vi "LED Shift Step.vi"(10 "LED Interpolate In":T1) -> (0 "Done":bool, 2 "LED Bit Array":u8[](array[numeric]), 3 "LED Interpolate Out":T1)   [LabVIEW 2014]
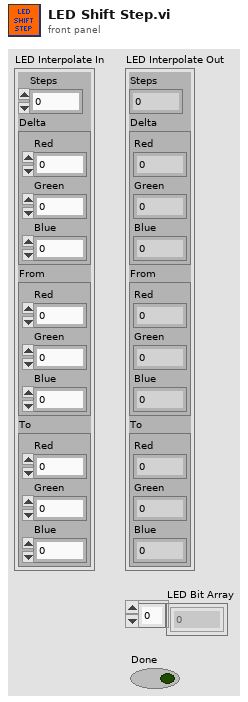
[diagram p1: front panel]
types:
  T1 = cluster{"Steps":i32, "Delta":cluster{"Red":dbl, "Green":dbl, "Blue":dbl}, "From":cluster{"Red":dbl, "Green":dbl, "Blue":dbl}, "To":cluster{"Red":dbl, "Green":dbl, "Blue":dbl}}
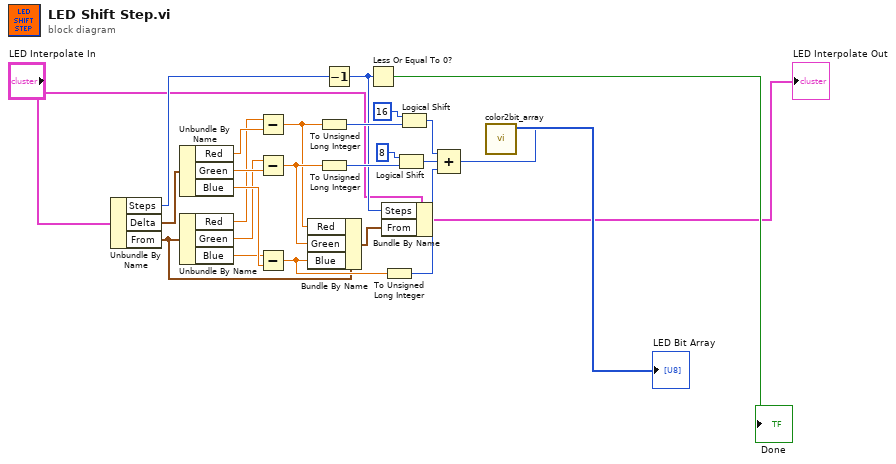
[diagram p0: block diagram]
diagram:
  n1 = Unbundle By Name("LED Interpolate In") -> ("Steps"=w3:i32, "Delta"=w7:cluster{"Red":dbl, "Green":dbl, "Blue":dbl}, "From"=w6:cluster{"Red":dbl, "Green":dbl, "Blue":dbl})
  n2 = Unbundle By Name(w7) -> ("Red"=w9:dbl, "Green"=w11:dbl, "Blue"=w13:dbl)
  n3 = Unbundle By Name(w6) -> ("Red"=w8:dbl, "Green"=w10:dbl, "Blue"=w12:dbl)
  n4 = Subtract(x=w8, y=w9) -> (x-y=w14:dbl)
  n5 = Subtract(x=w10, y=w11) -> (x-y=w20:dbl)
  n6 = Subtract(x=w12, y=w13) -> (x-y=w22:dbl)
  n7 = Bundle By Name(cluster=w6, "Red"=w14, "Green"=w20, "Blue"=w22) -> (w26:cluster{"Red":dbl, "Green":dbl, "Blue":dbl})
  n8 = To Unsigned Long Integer(number=w14) -> (unsigned 32bit integer=w15:u32)
  n9 = To Unsigned Long Integer(number=w20) -> (unsigned 32bit integer=w19:u32)
  n10 = Decrement(x=w3) -> (x-1=w4:i32)
  n11 = Less Or Equal To 0?(x=w4) -> (x <= 0?=→"Done":bool)
  n12 = Bundle By Name(cluster="LED Interpolate In", "Steps"=w4, "From"=w26) -> (→"LED Interpolate Out":T1)
  n13 = To Unsigned Long Integer(number=w22) -> (unsigned 32bit integer=w23:u32)
  n14 = Logical Shift(y=i16 8, x=w19) -> (x << y=w21:u32)
  n15 = Logical Shift(y=i16 16, x=w15) -> (x << y=w17:u32)
  n16 = Compound Arithmetic op=ADD(w17, w21, w23) -> (w24:u32)
  n17 = call "color2bit_array.vi"("Input Color"=w24) -> ("Bit Array"=→"LED Bit Array":u8[])  [unwired: 10 in]
